vi "Draw Background.vi"(7 "draw options":T2={"Background Color"=16777215, "Grid Color"=13816530, "Angle Units"=enum."Radians", "Draw Solid Background"=TRUE, "Draw Grid"=TRUE, "Grid Spacing"=1.0, "AutoScale"=TRUE, "Fit to Radius"=1.0, "data row options"=[]}, 9 "scaling info":T1={"pixels per unit"=1.0, "fit radius (units)"=1.0, "center point (pixels)"={"x"=0, "y"=0}}, 10 "DrawAreaSize":T5={"Width"=100, "Height"=100}, 11 "picture in":picture) -> (3 "picture out":picture)   [LabVIEW 2017, in "NI_Robotics_2D Rangefinder Picture.lvlib"]
uses:
  <vilib>/robotics/Controls/2D Rangefinder/2D Rangefinder Picture/NI_Robotics_2D Rangefinder Picture.lvlib
  <vilib>/Utility/miscctls.llb/LVBoundsTypeDef.ctl
  <vilib>/robotics/Controls/2D Rangefinder/2D Rangefinder Picture/Draw Options.ctl
  <vilib>/robotics/Controls/Utilities/Angle Units.ctl
  <vilib>/robotics/Controls/2D Rangefinder/2D Rangefinder Picture/Data Row Options.ctl
  <vilib>/robotics/Controls/2D Rangefinder/2D Rangefinder Picture/Scaling Info.ctl
  <vilib>/robotics/Controls/Utilities/NI_Robotics_Control Utilities.lvlib
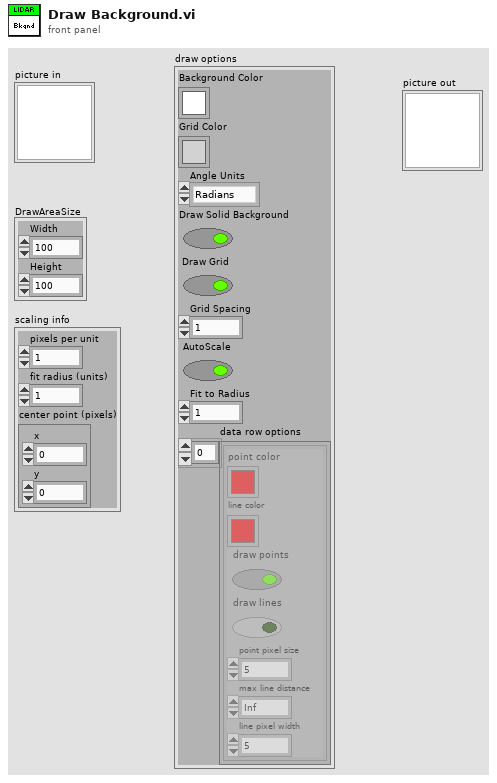
[diagram p1: front panel]
types:
  T1 = typedef "NI_Robotics_2D Rangefinder Picture.lvlib/Scaling Info.ctl" = cluster{"pixels per unit":dbl, "fit radius (units)":dbl, "center point (pixels)":cluster{"x":i16, "y":i16}}
  T2 = typedef "NI_Robotics_2D Rangefinder Picture.lvlib/Draw Options.ctl" = cluster{"Background Color":u32, "Grid Color":u32, "Angle Units":T3, "Draw Solid Background":bool, "Draw Grid":bool, "Grid Spacing":dbl, "AutoScale":bool, "Fit to Radius":dbl, "data row options":T4[]}
  T3 = typedef "NI_Robotics_Control Utilities.lvlib/Angle Units.ctl" = enum16{"Radians", "Degrees"}
  T4 = typedef "NI_Robotics_2D Rangefinder Picture.lvlib/Data Row Options.ctl" = cluster{"point color":u32, "line color":u32, "draw points":bool, "draw lines":bool, "point pixel size":u16, "max line distance":dbl, "line pixel width":u16}
  T5 = typedef "LVBoundsTypeDef.ctl" = cluster{"Width":u32, "Height":u32}
  T6 = cluster{"left":i16, "top":i16, "right":i16, "bottom":i16}
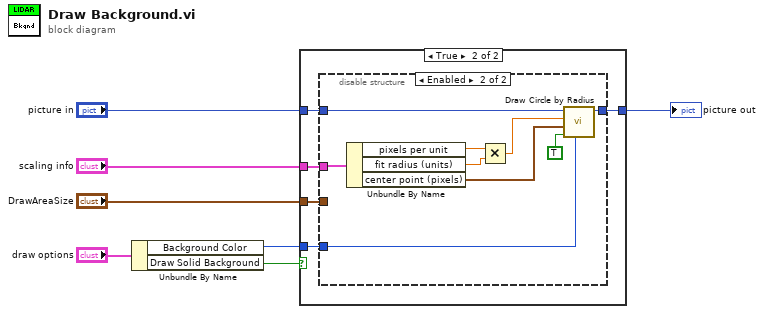
[diagram p0: block diagram]
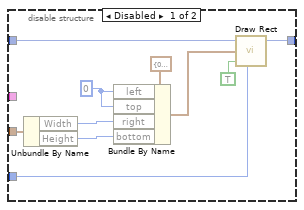
[diagram p3: hidden frame]
diagram:
  n1 = Unbundle By Name("draw options") -> ("Background Color"=w5:u32, "Draw Solid Background"=w6:bool)
  n2 = case shown="True" w6 {
    tunnel: w5 -> [_ w11]
    tunnel: "picture in" -> [w8 w13]
    tunnel: [w8 w12] -> w3
    tunnel: "DrawAreaSize" -> [_ w10]
    tunnel: "scaling info" -> [_ w9]
    frame False {
    }
    frame True {
      n3 = disable-structure shown="Enabled" {
        disable-tunnel: w13 -> [w23 w32]
        disable-tunnel: [w22 w25] -> w12
        disable-tunnel: w11 -> [w21 w29]
        disable-tunnel: w10 -> [w16 _]
        disable-tunnel: w9 -> [_ w31]
        frame Disabled {
          w18 = i16 0 ("left")
          n4 = Unbundle By Name(w16) -> ("Width"=w15:u32, "Height"=w14:u32)
          n5 = Bundle By Name(cluster=T6 {"left"=0, "top"=0, "right"=0, "bottom"=0} ("rect"), "left"=w18, "top"=w18, "right"=w15, "bottom"=w14) -> (w17:T6)
          n6 = call <vilib>:"Draw Rect.vi"("picture"=w23, "rect"=w17, "fill?(F)"=TRUE, "color(black)"=w21) -> ("new picture"=w22:picture)  [unwired: 5 in]
        }
        frame Enabled {
          n7 = Unbundle By Name(w31) -> ("pixels per unit"=w28:dbl, "fit radius (units)"=w27:dbl, "center point (pixels)"=w30:cluster{"x":i16, "y":i16})
          n8 = Multiply(x=w28, y=w27) -> (x*y=w26:dbl)
          n9 = call <vilib>:"Draw Circle by Radius.vi"("color(black)"=w29, "fill?(F)"=TRUE, "pixel center"=w30, "radius"=w26, "picture"=w32) -> ("new picture"=w25:picture)  [unwired: 6 in]
        }
      }
    }
  }
  "picture out" <- w3
